vi "newRunSAS.vi"(8 "error in":errorcluster, 11 "AirSAS Controls":T1={"Receive Duration"=0.0, "I/O"={"DAQmx Device"="Dev1", "AO Range"=0.0, "AI Range"=0.0, "DAQ Group Delay"=0.0, "Fs"=0.0}, "Hardware"={"Centerpos"=[], "TXpos"=[], "RX1pos"=[], "RX2pos"=[], "Angle"=0.0, "Height"=0.0}, "Waveform"={"LFM Parameters"={"Duration"=1.0, "Fstart (Hz)"=1000.0, "Fstop (Hz)"=10000.0, "Out. Amplitude (Vpk)"=1.0, "Window %"=10.0}, "Transmit Waveform"={"t0"=timestamp(0 s since 1904-01-01), "dt"=1.0, "Y"=[]}}, "LINX Resource"={"IO"=enum."Remote", "Interface"=enum."Serial", "LINX Device Config"={"Interface"=enum."Serial", "COM Port"="COM13", "TCP Configuration"={"IP Address"="", "Port"=0}, "Device Family"=1, "Device ID"=1, "Device Name"="myRIO-1900", "TCP Ref"=refnum, "Channels"={"DI"=[0, 1, 2, 3, 4, 5, 6, 7, 8, 9, 10, 11, 12, 13, 14, 15, 16, 17, 18, 19, 20, 21, 22, 23, 24, 25, 26, 27, 28, 29, 30, 31, 32, 33, 34, 35, 36, 37, 38, 39, 40, 41, 42, 43, 44, 45, 46], "DO"=[0, 1, 2, 3, 4, 5, 6, 7, 8, 9, 10, 11, 12, 13, 14, 15, 16, 17, 18, 19, 20, 21, 22, 23, 24, 25, 26, 27, 28, 29, 30, 31, 32, 33, 34, 35, 36, 37, 38, 39, 40, 41, 42, 43, 44, 45, 46], "AI"=[0, 1, 2, 3, 4, 5, 6, 7, 8, 9, 10, 11], "AO"=[], "PWM"=[3, 5, 6, 9, 10], "QE"=[], "UART"=[0, 1], "I2C 2"=[0], "SPI"=[0], "CAN"=[], "Servo"=[], "AI Ref (V)"=0.0, "AI Resolution (Bits)"=0, "AO Ref (V)"=0.0, "AO Resolution (Bits)"=0}}}, "Port"=3000.0} {"Waveform"."LFM Parameters"."Window %" format="%.2g"; "Waveform"."LFM Parameters"."Out. Amplitude (Vpk)" format="%0.2f"; "Waveform"."LFM Parameters"."Fstop (Hz)" format="%^.3e"; "Waveform"."LFM Parameters"."Fstart (Hz)" format="%^.3e"; "Waveform"."LFM Parameters"."Duration" format="%.3f"}) -> (0 "error out":errorcluster, 3 "AirSAS Controls 2":T1={"Receive Duration"=0.0, "I/O"={"DAQmx Device"="Dev1", "AO Range"=0.0, "AI Range"=0.0, "DAQ Group Delay"=0.0, "Fs"=0.0}, "Hardware"={"Centerpos"=[], "TXpos"=[], "RX1pos"=[], "RX2pos"=[], "Angle"=0.0, "Height"=0.0}, "Waveform"={"LFM Parameters"={"Duration"=1.0, "Fstart (Hz)"=1000.0, "Fstop (Hz)"=10000.0, "Out. Amplitude (Vpk)"=1.0, "Window %"=10.0}, "Transmit Waveform"={"t0"=timestamp(0 s since 1904-01-01), "dt"=1.0, "Y"=[]}}, "LINX Resource"={"IO"=enum."Remote", "Interface"=enum."Serial", "LINX Device Config"={"Interface"=enum."Serial", "COM Port"="COM13", "TCP Configuration"={"IP Address"="", "Port"=0}, "Device Family"=1, "Device ID"=1, "Device Name"="myRIO-1900", "TCP Ref"=refnum, "Channels"={"DI"=[0, 1, 2, 3, 4, 5, 6, 7, 8, 9, 10, 11, 12, 13, 14, 15, 16, 17, 18, 19, 20, 21, 22, 23, 24, 25, 26, 27, 28, 29, 30, 31, 32, 33, 34, 35, 36, 37, 38, 39, 40, 41, 42, 43, 44, 45, 46], "DO"=[0, 1, 2, 3, 4, 5, 6, 7, 8, 9, 10, 11, 12, 13, 14, 15, 16, 17, 18, 19, 20, 21, 22, 23, 24, 25, 26, 27, 28, 29, 30, 31, 32, 33, 34, 35, 36, 37, 38, 39, 40, 41, 42, 43, 44, 45, 46], "AI"=[0, 1, 2, 3, 4, 5, 6, 7, 8, 9, 10, 11], "AO"=[], "PWM"=[3, 5, 6, 9, 10], "QE"=[], "UART"=[0, 1], "I2C 2"=[0], "SPI"=[0], "CAN"=[], "Servo"=[], "AI Ref (V)"=0.0, "AI Resolution (Bits)"=0, "AO Ref (V)"=0.0, "AO Resolution (Bits)"=0}}}, "Port"=3000.0} {"Waveform"."LFM Parameters"."Window %" format="%.2g"; "Waveform"."LFM Parameters"."Out. Amplitude (Vpk)" format="%0.2f"; "Waveform"."LFM Parameters"."Fstop (Hz)" format="%^.3e"; "Waveform"."LFM Parameters"."Fstart (Hz)" format="%^.3e"; "Waveform"."LFM Parameters"."Duration" format="%.3f"})   [LabVIEW 2018]
uses:
  N:/SRDD-Student/Ng/fromTom/Air SAS Data Acquisition/controls/Air SAS Controls.ctl
  <vilib>/MakerHub/LINX/Private/Type Defs/LINX Ref.ctl
  <vilib>/MakerHub/LINX/Private/Type Defs/Platform.ctl
  <vilib>/MakerHub/LINX/Private/Type Defs/Interface.ctl
  <vilib>/MakerHub/LINX/Private/Device/Type Defs/LINX Device Config.ctl
  <vilib>/MakerHub/LINX/Private/Device/Type Defs/TCP Config.ctl
  <vilib>/MakerHub/LINX/Private/Device/Type Defs/Channels.ctl
  <vilib>/Analysis/4window.llb/Cosine Tapered Window (DBL).vi
  <vilib>/Waveform/WDTOps.llb/WDT Number of Waveform Samples DBL.vi
  <vilib>/regexp/Match Regular Expression.xnode
  <vilib>/Analysis/NI_AALBase.lvlib
  <vilib>/Analysis/NI_AALPro.lvlib
  <vilib>/MakerHub/LINX/LMH-LINX.lvlib
  <vilib>/MakerHub/LINX/Private/Device/Device.lvlib
panel:
  in  "Folder Path":path=path "C:/Users/jqn5303/Desktop/testfiles"
  in  "stop":bool
  out "Transmit Waveform":waveform(dbl)(graph)
  in  "LFM Parameters":T8={"Fs (Hz)"=100000.0, "Sweep Length (s)"=0.001, "Fstart (Hz)"=10000.0, "Fstop (Hz)"=10000.0, "Out. Amplitude (Vpk)"=1.0, "Window %"=10.0} {"Window %" format="%.2g"; "Out. Amplitude (Vpk)" format="%0.2f"; "Fstop (Hz)" format="%^.3e"; "Fstart (Hz)" format="%^.3e"; "Sweep Length (s)" format="%.3f"; "Fs (Hz)" min=1000.0 max=2000000.0 format="%^.0e"}
  in  "Generate LFM":bool
  in  "Start Acquisition":bool
  out "Acquired Data":waveform(dbl)(graph)
  out "Slide":cluster{dbl, dbl, dbl}(slide)={0.0, 227.2365805168986, 42.94234592445328} scale=0.0..900.0
  out "Gauge":cluster{dbl, dbl, dbl}(knob)={0.0, -178.0803549193409, -96.36742372843878} scale format="%#_g°"
  in  "Motion Control":T9={"SAS Geometry"=enum."Circular", "Angular Step"=1.0, "Vertical Step"=0.0, "Vertical Min"=0.0, "Vertical Max"=0.0, "Angular Start"=0.0, "Angular Stop"=359.0}
  in  "Receive Duration":dbl=0.01
  in  "Averages":dbl=1.0 min=1.0 step=1.0
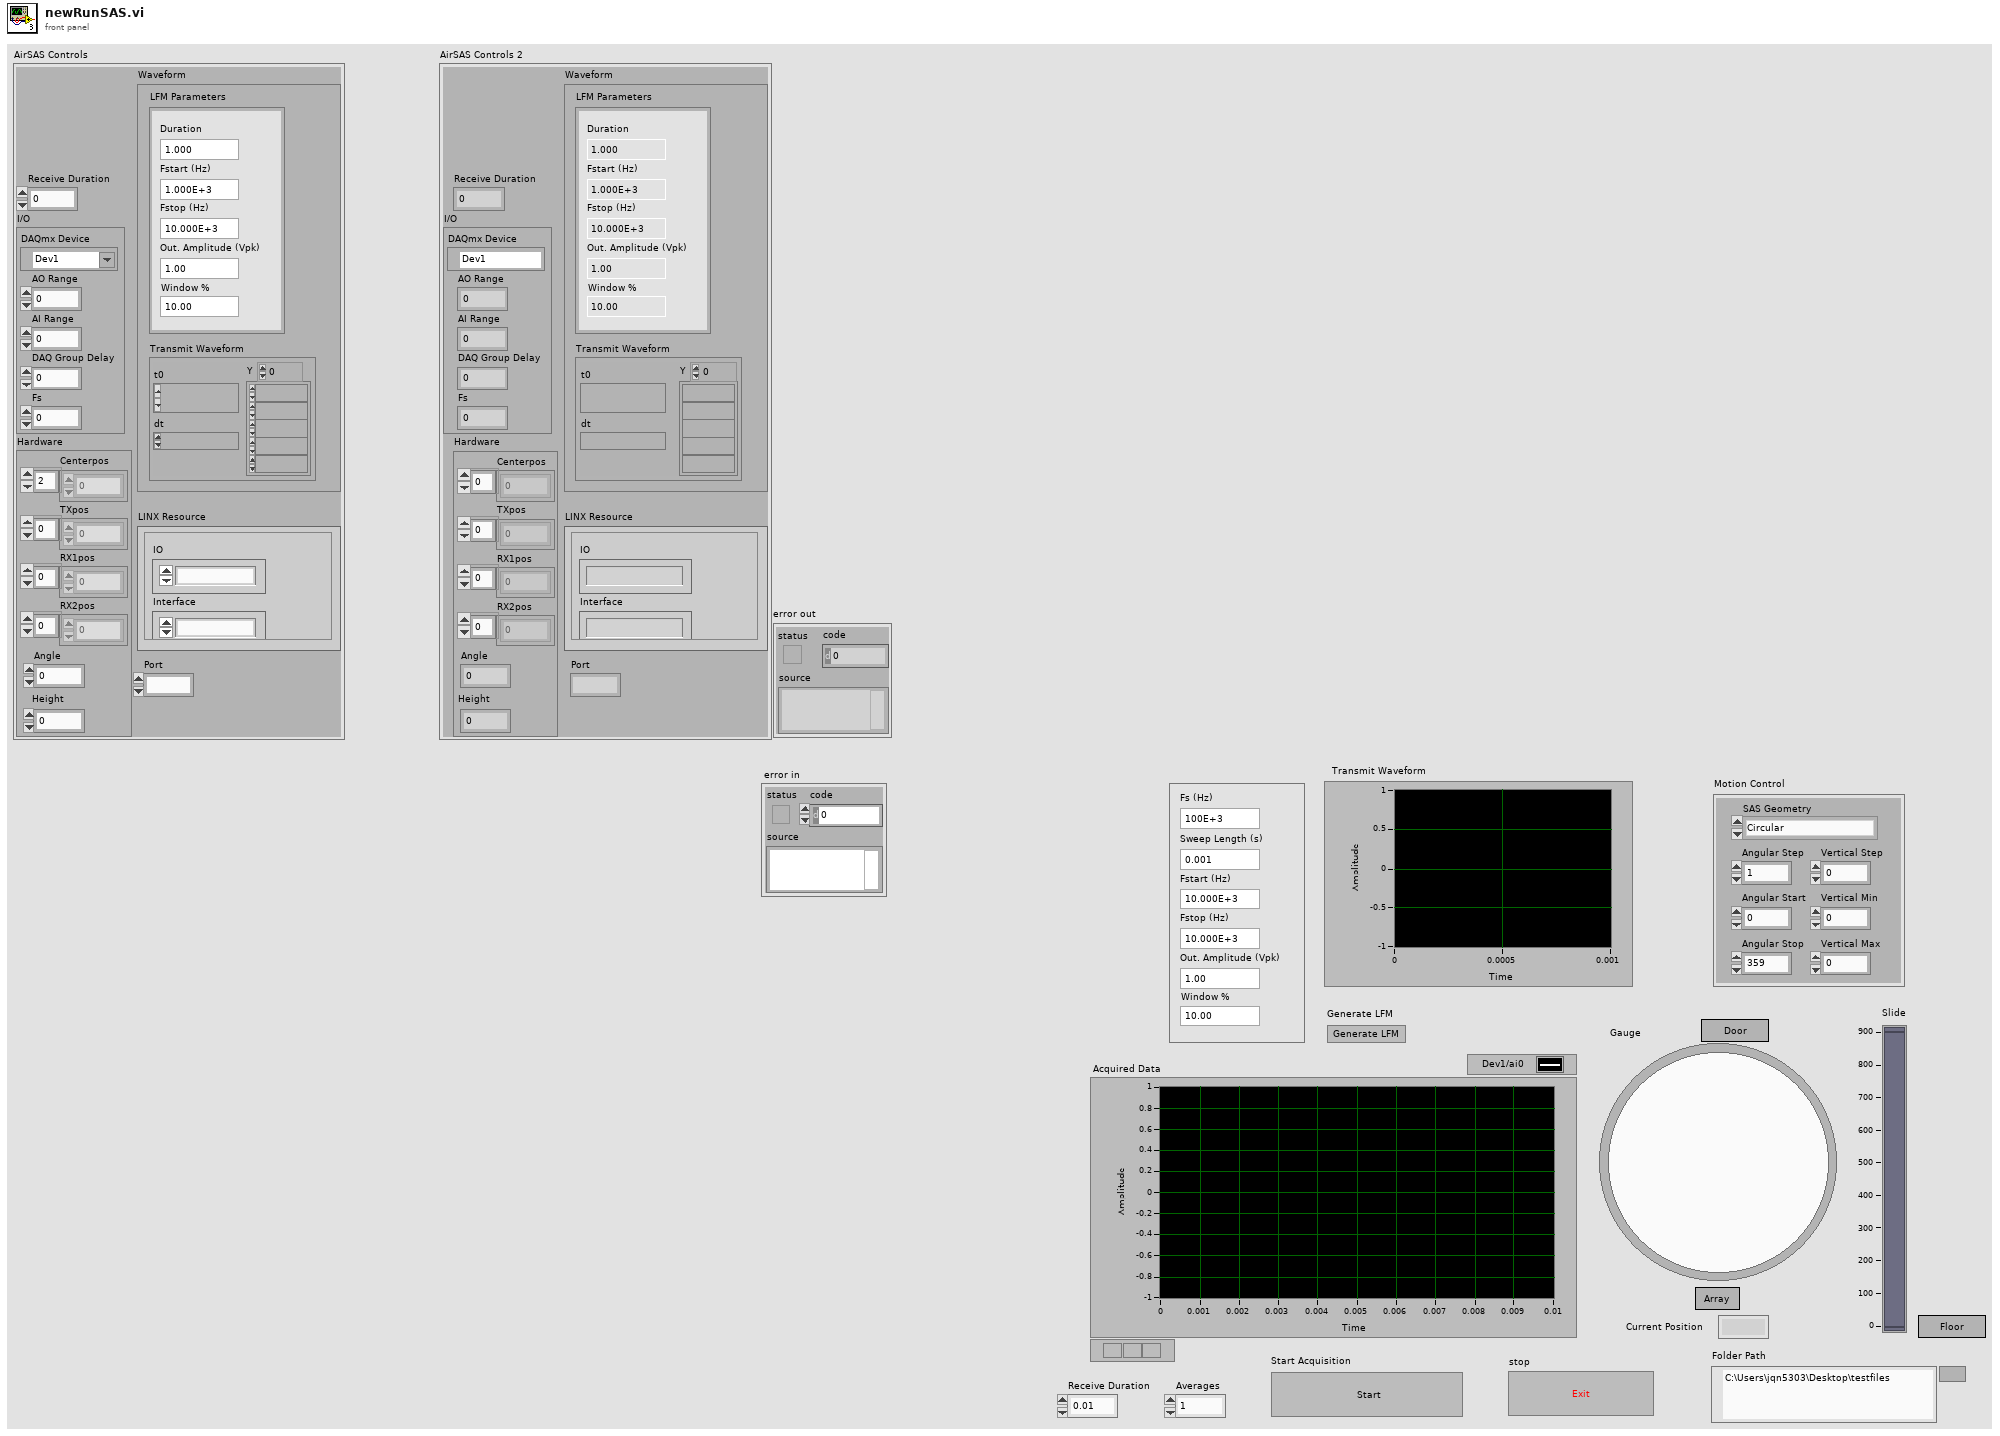
[diagram p1: front panel]
types:
  T1 = typedef "Air SAS Controls.ctl" = cluster{"Receive Duration":dbl, "I/O":cluster{"DAQmx Device":tag, "AO Range":dbl, "AI Range":dbl, "DAQ Group Delay":dbl, "Fs":dbl}, "Hardware":cluster{"Centerpos":dbl[], "TXpos":dbl[], "RX1pos":dbl[], "RX2pos":dbl[], "Angle":dbl, "Height":dbl}, "Waveform":cluster{"LFM Parameters":cluster{"Duration":dbl, "Fstart (Hz)":dbl, "Fstop (Hz)":dbl, "Out. Amplitude (Vpk)":dbl, "Window %":dbl}, "Transmit Waveform":waveform(dbl)}, "LINX Resource":T2, "Port":dbl}
  T2 = typedef "LMH-LINX.lvlib/LINX Ref.ctl" = cluster{"IO":T3, "Interface":T4, "LINX Device Config":T5}
  T3 = typedef "LMH-LINX.lvlib/Platform.ctl" = enum16{"Remote", "Local"}
  T4 = typedef "LMH-LINX.lvlib/Interface.ctl" = enum16{"Serial", "TCP"}
  T5 = typedef "LMH-LINX.lvlib/Device.lvlib/LINX Device Config.ctl" = cluster{"Interface":T4, "COM Port":refnum<visa-resource-name>, "TCP Configuration":T6, "Device Family":u8, "Device ID":u8, "Device Name":string, "TCP Ref":refnum<k5>, "Channels":T7}
  T6 = typedef "LMH-LINX.lvlib/Device.lvlib/TCP Config.ctl" = cluster{"IP Address":string, "Port":u16}
  T7 = typedef "LMH-LINX.lvlib/Channels.ctl" = cluster{"DI":u8[], "DO":u8[], "AI":u8[], "AO":u8[], "PWM":u8[], "QE":u8[], "UART":u8[], "I2C 2":u8[], "SPI":u8[], "CAN":u8[], "Servo":u8[], "AI Ref (V)":dbl, "AI Resolution (Bits)":u8, "AO Ref (V)":dbl, "AO Resolution (Bits)":u8}
  T8 = cluster{"Fs (Hz)":dbl, "Sweep Length (s)":dbl, "Fstart (Hz)":dbl, "Fstop (Hz)":dbl, "Out. Amplitude (Vpk)":dbl, "Window %":dbl}
  T9 = cluster{"SAS Geometry":enum16{"Circular", "Cylindrical", "Spiral"}, "Angular Step":dbl, "Vertical Step":dbl, "Vertical Min":dbl, "Vertical Max":dbl, "Angular Start":dbl, "Angular Stop":dbl}
  T10 = enum8{"Enabled", "Disabled", "Disabled and Grayed Out"}
  T11 = cluster{"Angular Start":dbl, dbl, "Angular Stop":dbl}
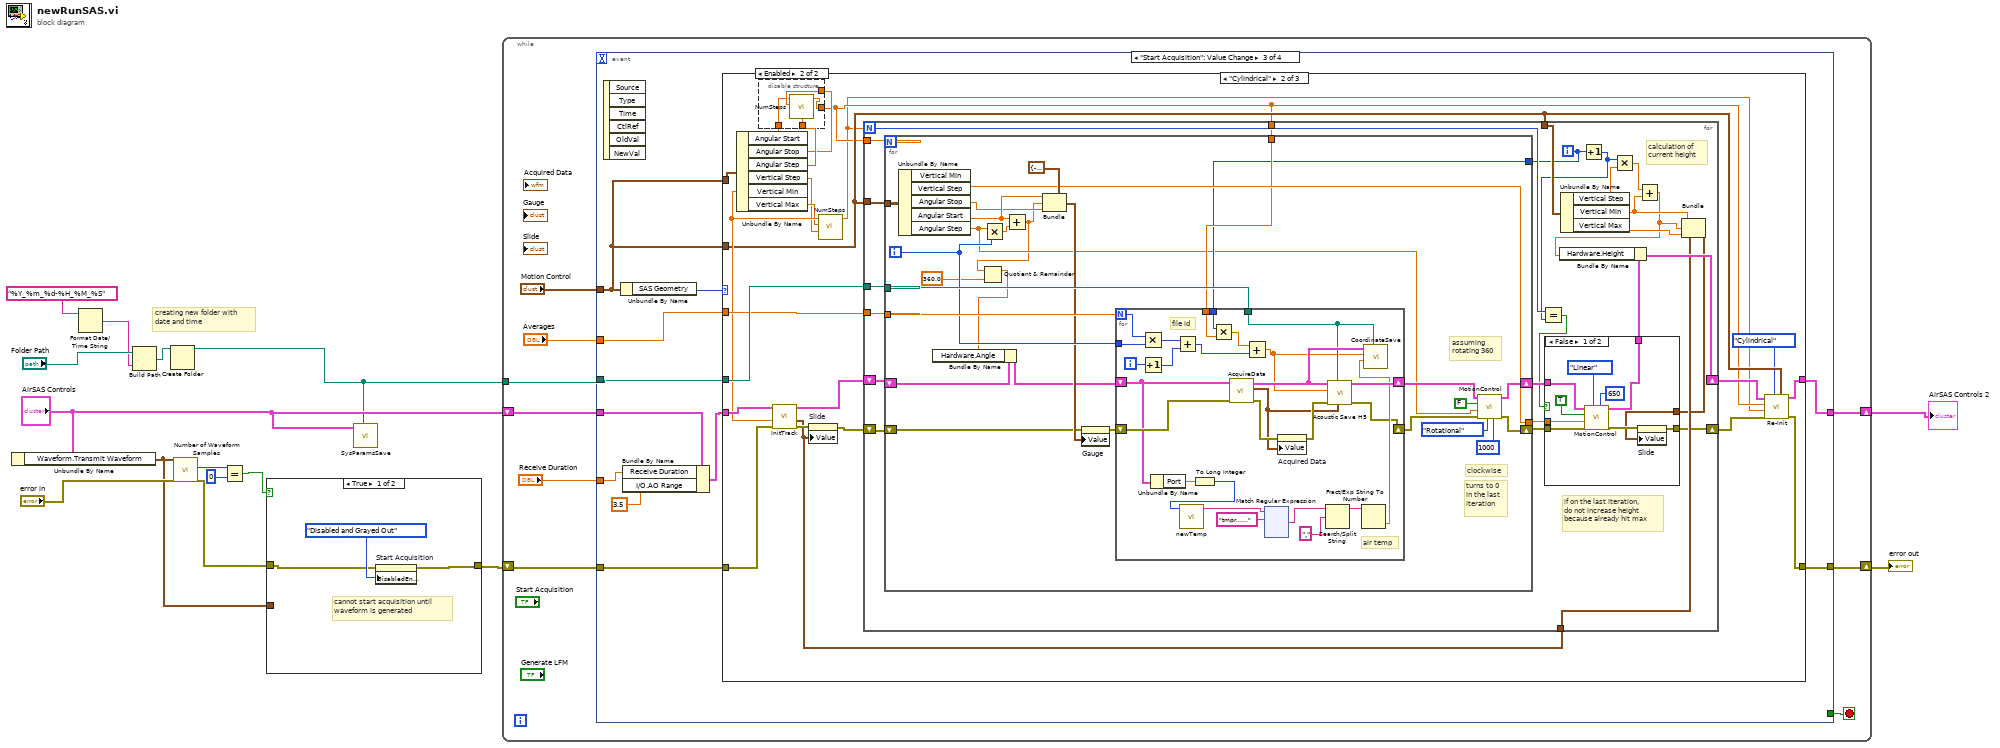
[diagram p0: block diagram]
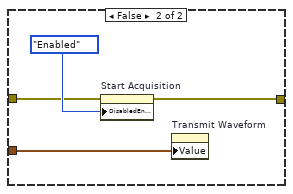
[diagram p2: hidden frame]
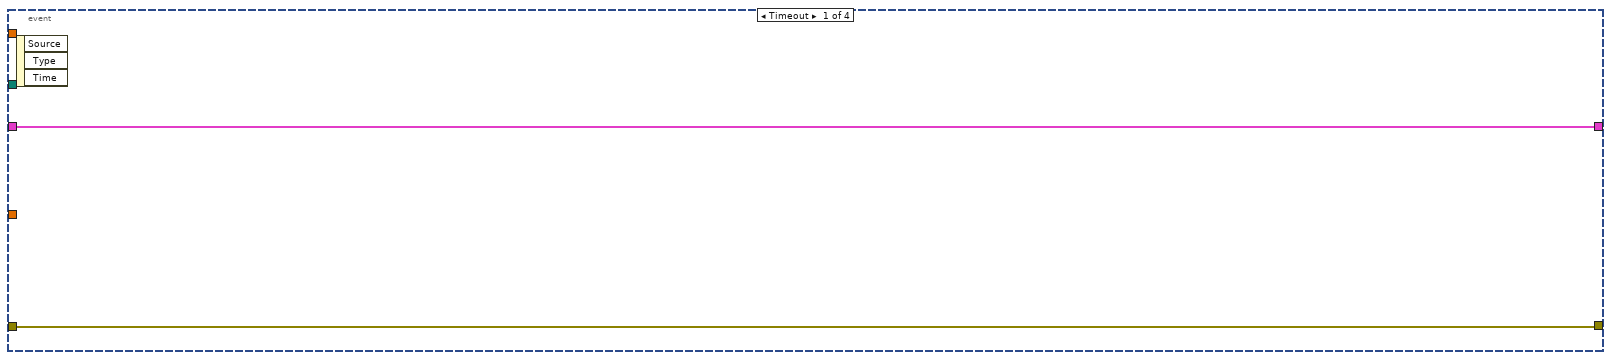
[diagram p3: hidden frame]
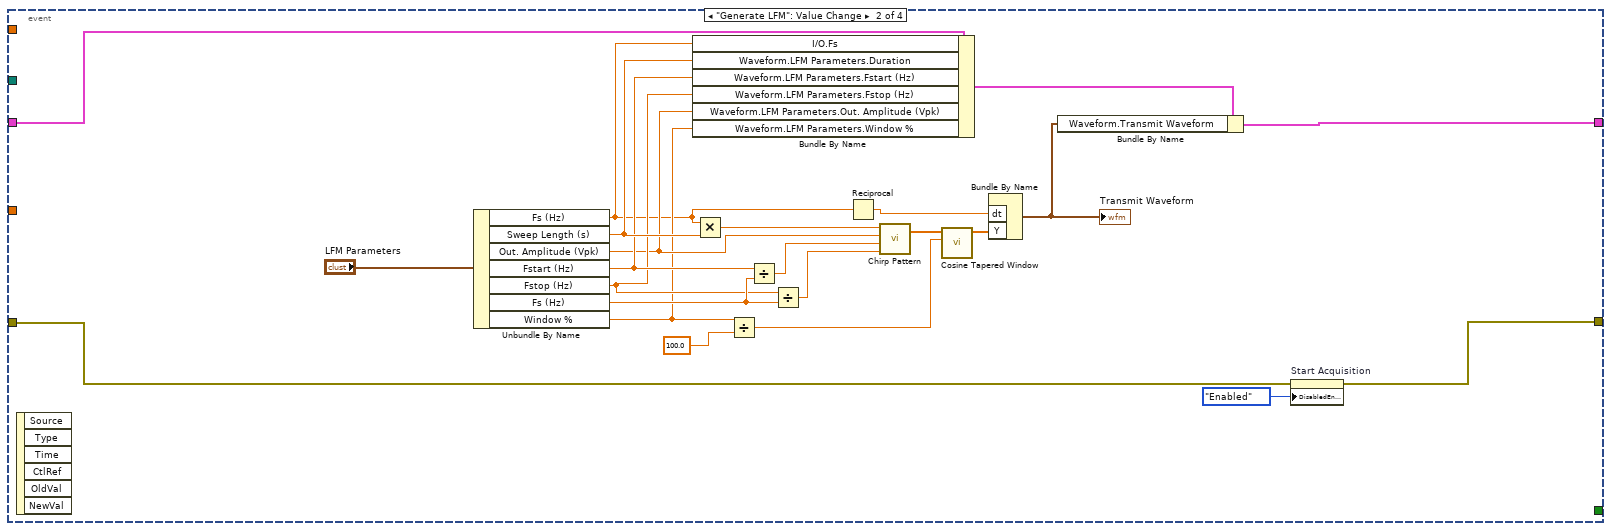
[diagram p4: hidden frame]
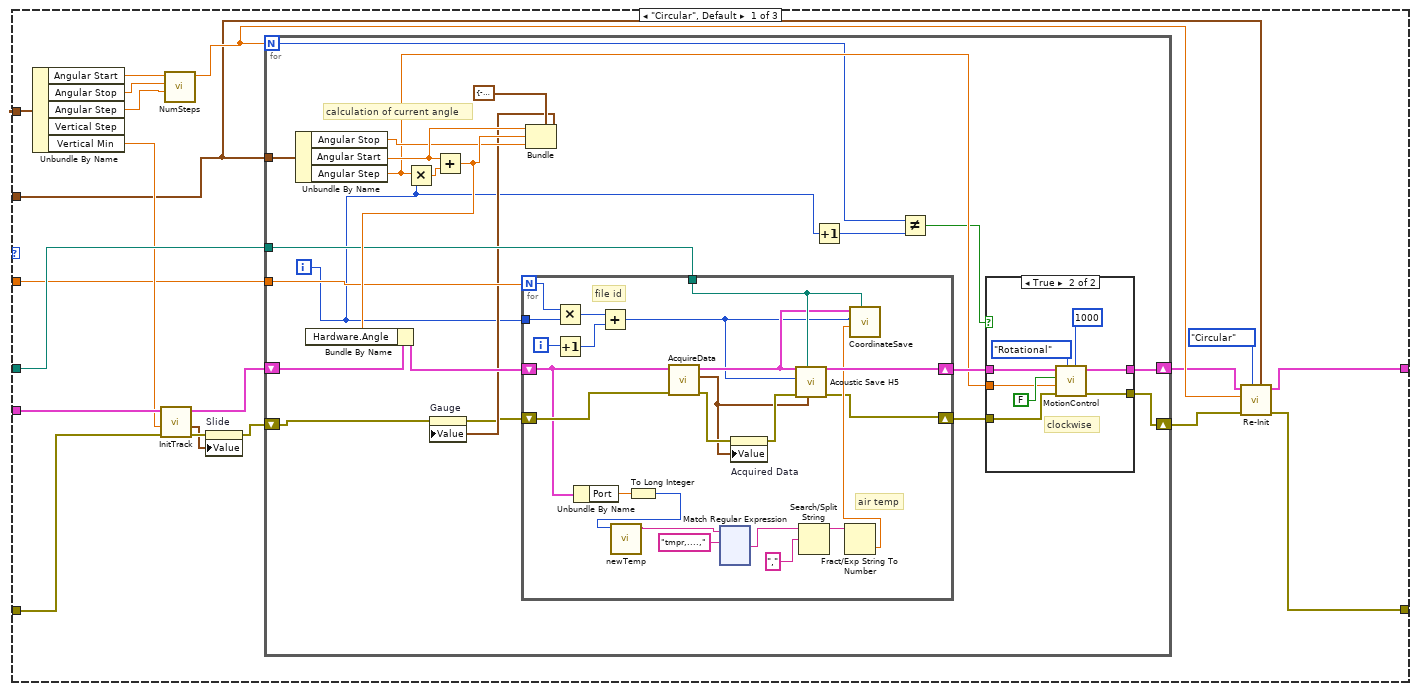
[diagram p5: hidden frame]
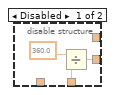
[diagram p7: hidden frame]
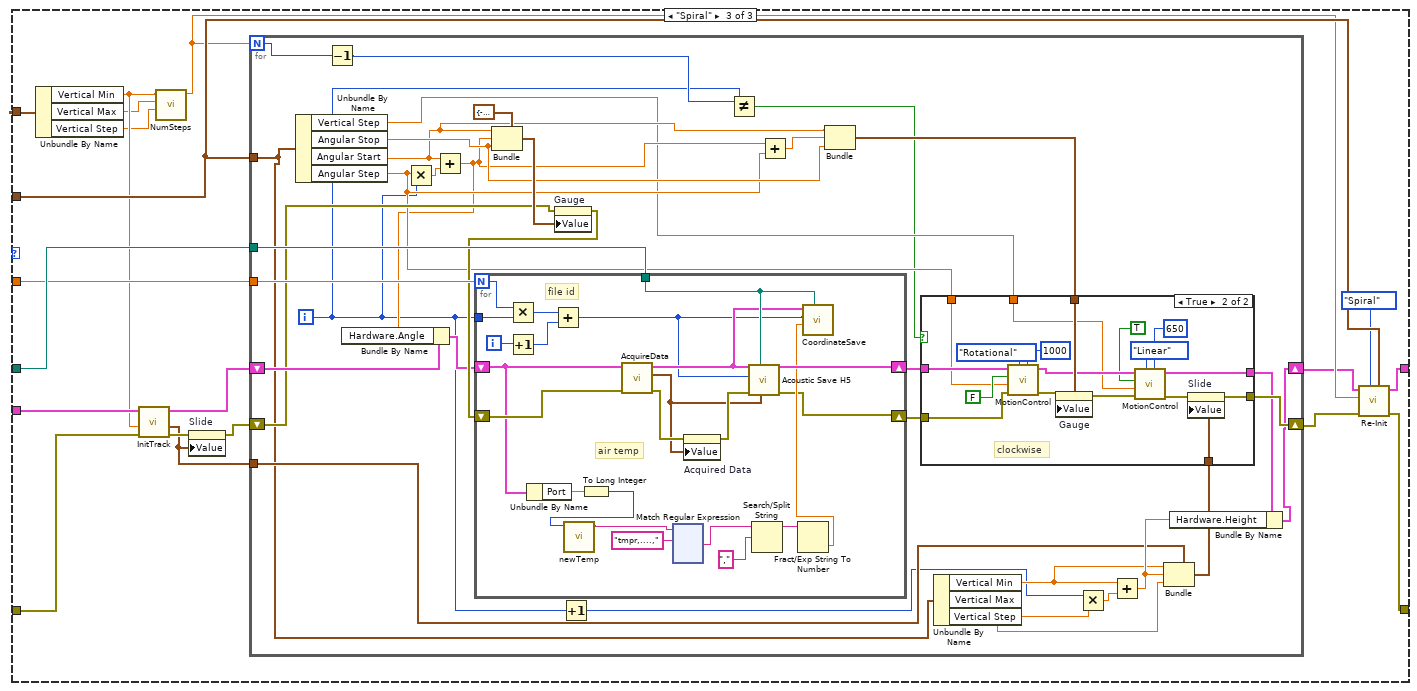
[diagram p9: hidden frame]
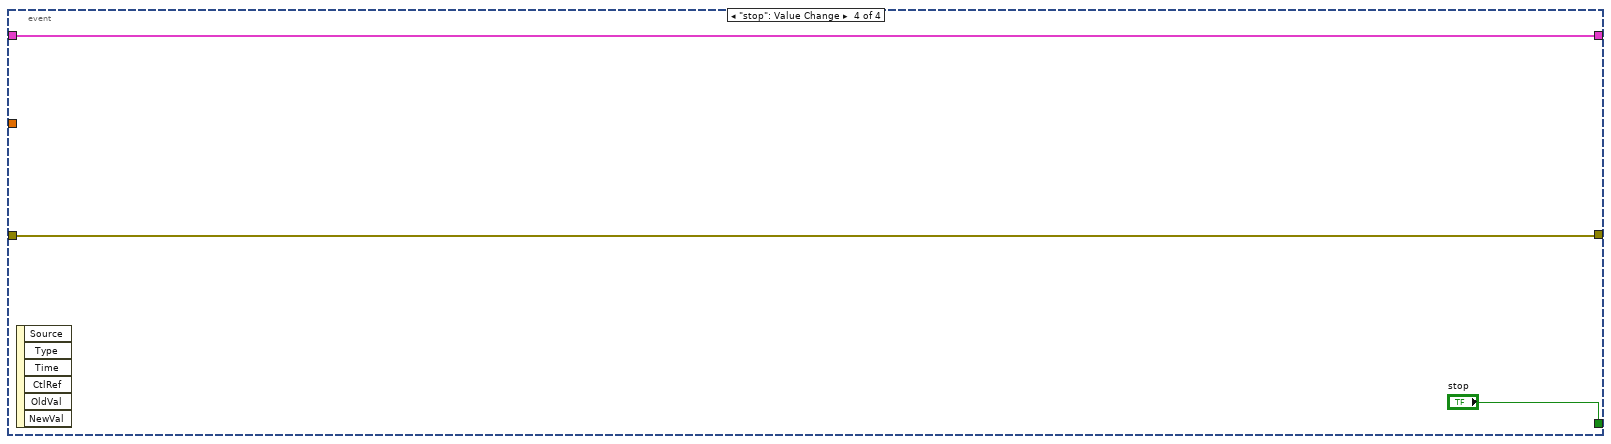
[diagram p11: hidden frame]
diagram:
  # "creating new folder with\ndate and time"
  n1 = Unbundle By Name("AirSAS Controls") -> ("Waveform.Transmit Waveform"=w8:waveform(dbl))
  n2 = Format Date/Time String(time format string (%c)="%Y_%m_%d-%H_%M_%S") -> (date/time string=w3:string)  [unwired: 2 in]
  n3 = Build Path(base path="Folder Path", name or relative path=w3) -> (appended path=w2:path)
  n4 = Create Folder(path (use dialog)=w2) -> (created path=w1:path)  [unwired: 2 in, 2 out]
  n5 = call-poly <vilib>:"Number of Waveform Samples.vi"("error in (no error)"="error in", "waveform in"=w8) -> ("error out"=w9:errorcluster, "number of samples"=w14:i32)  [unwired: 7 in, 1 out]
  n6 = Equal?(x=w14, y=0) -> (x = y?=w12:bool)
  n7 = case shown="True" w12 {
    tunnel: [w16 w20] -> w10
    tunnel: w9 -> [w17 w19]
    tunnel: w8 -> [_ w21]
    frame True {
      # "cannot start acquisition until\nwaveform is generated"
      n8 = property on="Start Acquisition" class="Bool"(error in=w17, "DisabledEnum"=T10."Disabled and Grayed Out" ("Disabled")) -> (error out=w16:errorcluster)  [unwired: 1 in, 1 out]
    }
    frame False {
      n9 = property on="Start Acquisition" class="Bool"(error in=w19, "DisabledEnum"=T10."Enabled" ("Disabled")) -> (error out=w20:errorcluster)  [unwired: 1 in, 1 out]
      n10 = property on="Transmit Waveform" class="WFGraph (strict)"("Value"=w21) -> ()  [unwired: 2 in, 2 out]
    }
  }
  n11 = call "SysParamsSave.vi"("Path"=w1, "AirSAS Controls"="AirSAS Controls") -> ()  [unwired: 10 in]
  n12 = while {
    shift-right: [w30] -> w7
    shift-left: "AirSAS Controls" -> [w31]
    shift-right: [w27] -> w15
    shift-left: w10 -> [w28]
    tunnel: w1 -> [w26]
    stop <- w29 stop-if-true
    n13 = event shown="[2] \"Start Acquisition\": Value Change" {
      selector: _ -> [_ _ _ _]
      dyn-events: _ -> [_ _ _ _]
      timeout: _ -> [_ _ _ _]
      tunnel: w31 -> [w33 w46 w64 w700]
      tunnel: [w33 w38 w59 w700] -> w30
      tunnel: [_ _ _ "stop"] -> w29
      tunnel: w28 -> [w32 w35 w63 w699]
      tunnel: [w32 w34 w58 w699] -> w27
      tunnel: w26 -> [_ _ w61 _]
      tunnel: "Motion Control" -> [_ _ w62 _]
      tunnel: "Receive Duration" -> [_ _ w66 _]
      tunnel: "Averages" -> [_ _ w60 _]
      event Timeout {
        n14 = event-data() -> ()  [unwired: 1 in, 3 out]
      }
      event "Generate LFM": Value Change {
        n15 = event-data() -> ()  [unwired: 1 in, 6 out]
        n16 = Unbundle By Name("LFM Parameters") -> ("Fs (Hz)"=w37:dbl, "Sweep Length (s)"=w45:dbl, "Out. Amplitude (Vpk)"=w42:dbl, "Fstart (Hz)"=w44:dbl, "Fstop (Hz)"=w43:dbl, "Fs (Hz)"=w54:dbl, "Window %"=w41:dbl)
        n17 = Bundle By Name(cluster=w46, "I/O.Fs"=w37, "Waveform.LFM Parameters.Duration"=w45, "Waveform.LFM Parameters.Fstart (Hz)"=w44, "Waveform.LFM Parameters.Fstop (Hz)"=w43, "Waveform.LFM Parameters.Out. Amplitude (Vpk)"=w42, "Waveform.LFM Parameters.Window %"=w41) -> (w40:T1)
        n18 = Multiply(x=w37, y=w45) -> (x*y=w56:dbl)
        n19 = Divide(x=w41, y=100.0) -> (x/y=w49:dbl)
        n20 = Divide(x=w44, y=w54) -> (x/y=w55:dbl)
        n21 = Divide(x=w43, y=w54) -> (x/y=w53:dbl)
        n22 = Reciprocal(x=w37) -> (1/x=w50:dbl)
        n23 = call <vilib>:"Chirp Pattern.vi"("f2"=w53, "f1"=w55, "amplitude"=w42, "samples"=w56) -> ("Chirp Pattern"=w52:dbl[])  [unwired: 1 out]
        n24 = call-poly <vilib>:"Cosine Tapered Window.vi"("ratio"=w49, "X"=w52) -> ("Windowed X"=w51:dbl[])  [unwired: 8 in, 1 out]
        n25 = Bundle By Name("dt"=w50, "Y"=w51) -> (w39:waveform(dbl))  [unwired: 1 in]
        "Transmit Waveform" <- w39
        n26 = Bundle By Name(cluster=w40, "Waveform.Transmit Waveform"=w39) -> (w38:T1)
        n27 = property on="Start Acquisition" class="Bool"(error in=w35, "DisabledEnum"=T10."Enabled" ("Disabled")) -> (error out=w34:errorcluster)  [unwired: 1 in, 1 out]
      }
      event "Start Acquisition": Value Change {
        n28 = event-data() -> ()  [unwired: 1 in, 6 out]
        n29 = Unbundle By Name(w62) -> ("SAS Geometry"=w67:enum16{"Circular", "Cylindrical", "Spiral"})
        n30 = Bundle By Name(cluster=w64, "Receive Duration"=w66, "I/O.AO Range"=3.5) -> (w57:T1)
        n31 = case shown="\"Cylindrical\"" w67 {
          tunnel: w62 -> [w87 w278 w508]
          tunnel: w57 -> [w85 w276 w506]
          tunnel: w63 -> [w83 w275 w505]
          tunnel: w62 -> [w76 w261 w500]
          tunnel: w61 -> [w86 w277 w507]
          tunnel: [w72 w262 w491] -> w59
          tunnel: w60 -> [w81 w273 w503]
          tunnel: [w74 w259 w498] -> w58
          frame "Circular", Default {
            n32 = Unbundle By Name(w87) -> ("Angular Start"=w71:dbl, "Angular Stop"=w70:dbl, "Angular Step"=w69:dbl, "Vertical Min"=w84:dbl)  [unwired: 1 out]
            n33 = call "InitTrack.vi"("AirSAS Controls in"=w85, "Vertical Min"=w84, "error in (no error)"=w83) -> ("AirSAS Controls out"=w82:T1, "output cluster"=w78:cluster{dbl, dbl, dbl}, "error out"=w80:errorcluster)  [unwired: 4 in]
            n34 = call "NumSteps.vi"("Step"=w69, "Stop"=w70, "Start"=w71) -> ("Numeric"=w77:dbl)  [unwired: 8 in]
            n35 = property on="Slide" class="Slide (strict)"(error in=w80, "Value"=w78) -> (error out=w79:errorcluster)  [unwired: 1 in, 1 out]
            n36 = for {
              N: w77 -> [w88]
              tunnel: w76 -> [w109]
              tunnel: w86 -> [w102]
              shift-right: [w98] -> w73
              shift-left: w82 -> [w108]
              tunnel: w81 -> [w101]
              shift-right: [w93] -> w75
              shift-left: w79 -> [w95]
              i -> [w89]
              # "calculation of current angle"
              n37 = Unbundle By Name(w109) -> ("Angular Stop"=w104:dbl, "Angular Start"=w106:dbl, "Angular Step"=w97:dbl)
              n38 = Multiply(x=w97, y=w89) -> (x*y=w107:dbl)
              n39 = Add(x=w106, y=w107) -> (x+y=w105:dbl)
              n40 = Bundle By Name(cluster=w108, "Hardware.Angle"=w105) -> (w100:T1)
              n41 = Bundle(cluster=cluster{dbl, dbl, dbl} {-172.55422153679154, 17.21837893351085, -51.118830131082746} ("Gauge 2"), w106, w105, w104) -> (w96:cluster{dbl, dbl, dbl})
              n42 = property on="Gauge" class="Knob (strict)"(error in=w95, "Value"=w96) -> (error out=w94:errorcluster)  [unwired: 1 in, 1 out]
              n43 = for {
                N: w101 -> [w139]
                tunnel: w89 -> [w138]
                tunnel: w102 -> [w124]
                shift-right: [w123] -> w99
                shift-left: w100 -> [w125]
                shift-right: [w120] -> w92
                shift-left: w94 -> [w136]
                i -> [w137]
                # "air temp"
                # "file id"
                n44 = Multiply(x=w139, y=w138) -> (x*y=w141:i32)
                n45 = Increment(x=w137) -> (x+1=w140:i32)
                n46 = Unbundle By Name(w125) -> ("Port"=w131:dbl)
                n47 = Add(x=w141, y=w140) -> (x+y=w122:i32)
                n48 = To Long Integer(number=w131) -> (32bit integer=w132:i32)
                n49 = call "newTemp.vi"("port"=w132) -> ("Response String"=w130:string)  [unwired: 10 in]
                n50 = call "AcquireData.vi"("error in"=w136, "AirSAS Controls In"=w125) -> ("error out"=w135:errorcluster, "data"=w133:waveform(dbl), "AirSAS Controls Out"=w123:T1)  [unwired: 7 in]
                n51 = xnode "Match Regular Expression"("input string"=w130, "regular expression"="tmpr,....,") -> ("after match"=w128:string)  [unwired: 4 in, 4 out]
                n52 = property on="Acquired Data" class="WFGraph (strict)"(error in=w135, "Value"=w133) -> (error out=w134:errorcluster)  [unwired: 1 in, 1 out]
                n53 = call "Acoustic Save H5.vi"("Captured Data"=w133, "base path"=w124, "error in (no error)"=w134, "ID"=w122) -> ("error out"=w120:errorcluster)  [unwired: 7 in]
                n54 = Search/Split String(string=w128, search string/char (-)=",") -> (substring before match=w129:string)  [unwired: 1 in, 2 out]
                n55 = Fract/Exp String To Number(string=w129) -> (number=w121:dbl)  [unwired: 3 in, 1 out]
                n56 = call "CoordinateSave.vi"("Path"=w124, "Air Temperature"=w121, "Flight"=w122, "AirSAS Controls"=w123) -> ()  [unwired: 8 in]
              }
              n57 = Increment(x=w89) -> (x+1=w90:i32)
              n58 = Not Equal?(x=w88, y=w90) -> (x != y?=w91:bool)
              n59 = case shown="True" w91 {
                tunnel: w99 -> [w111 w117]
                tunnel: [w111 w116] -> w98
                tunnel: w97 -> [_ w114]
                tunnel: [w110 w113] -> w93
                tunnel: w92 -> [w110 w112]
                frame False {
                }
                frame True {
                  # "clockwise"
                  n60 = call "MotionControl.vi"("Frequency (Hz) 3"=u32 1000, "Motion Type"=enum16{"Linear", "Rotational"}."Rotational", "Error In"=w112, "Distance"=w114, "Direction"=FALSE, "AirSAS Controls"=w117) -> ("Error Out"=w113:errorcluster, "output cluster"=w116:T1)  [unwired: 4 in]
                }
              }
            }
            n61 = call "Re-Init.vi"("Motion Control"=w76, "Enum"=enum16{"Circular", "Cylindrical", "Spiral"}."Circular", "error in (no error)"=w75, "# rot. steps"=w77, "AirSAS Controls"=w73) -> ("error out"=w74:errorcluster, "output cluster"=w72:T1)  [unwired: 5 in]
          }
          frame "Cylindrical" {
            n62 = Unbundle By Name(w278) -> ("Angular Start"=w264:dbl, "Angular Stop"=w265:dbl, "Angular Step"=w272:dbl, "Vertical Step"=w266:dbl, "Vertical Min"=w268:dbl, "Vertical Max"=w267:dbl)
            n63 = disable-structure shown="Enabled" {
              disable-tunnel: w272 -> [w280 w285]
              disable-tunnel: [w279 w282] -> w258
              disable-tunnel: w265 -> [_ w284]
              disable-tunnel: w264 -> [_ w283]
              frame Disabled {
                n64 = Divide(x=360.0, y=w280) -> (x/y=w279:dbl)
              }
              frame Enabled {
                n65 = call "NumSteps.vi"("Step"=w285, "Stop"=w284, "Start"=w283) -> ("Numeric"=w282:dbl)  [unwired: 8 in]
              }
            }
            n66 = call "InitTrack.vi"("AirSAS Controls in"=w276, "Vertical Min"=w268, "error in (no error)"=w275) -> ("AirSAS Controls out"=w274:T1, "output cluster"=w269:cluster{dbl, dbl, dbl}, "error out"=w271:errorcluster)  [unwired: 4 in]
            n67 = property on="Slide" class="Slide (strict)"(error in=w271, "Value"=w269) -> (error out=w270:errorcluster)  [unwired: 1 in, 1 out]
            n68 = call "NumSteps.vi"("Step"=w266, "Stop"=w267, "Start"=w268) -> ("Numeric"=w257:dbl)  [unwired: 8 in]
            n69 = for {
              N: w257 -> [w290]
              tunnel: w261 -> [w310]
              tunnel: w277 -> [w307]
              shift-right: [w299] -> w263
              shift-left: w274 -> [w309]
              tunnel: w273 -> [w306]
              tunnel: w258 -> [w305]
              tunnel: w261 -> [w302]
              tunnel: w269 -> [w298]
              shift-right: [w294] -> w260
              shift-left: w270 -> [w308]
              tunnel: w258 -> [w287]
              i -> [w286]
              # "if on the last iteration,\ndo not increase height\nbecause already hit max"
              # "calculation of\ncurrent height"
              n70 = for {
                N: w305 -> [_]
                tunnel: w310 -> [w349]
                tunnel: w307 -> [w343]
                tunnel: w306 -> [w342]
                shift-right: [w327] -> w293
                shift-left: w309 -> [w348]
                shift-right: [w329] -> w304
                shift-left: w308 -> [w334]
                tunnel: [w340] -> w303
                tunnel: w287 -> [w338]
                tunnel: w286 -> [w337]
                i -> [w339]
                # "assuming\nrotating 360"
                # "turns to 0\nin the last\niteration"
                # "clockwise"
                n71 = Unbundle By Name(w349) -> ("Vertical Step"=w340:dbl, "Angular Stop"=w345:dbl, "Angular Start"=w346:dbl, "Angular Step"=w326:dbl)  [unwired: 1 out]
                n72 = Multiply(x=w326, y=w339) -> (x*y=w347:dbl)
                n73 = Add(x=w346, y=w347) -> (x+y=w325:dbl)
                n74 = Quotient & Remainder(x=w325, y=360.0) -> (x-y*floor(x/y)=w323:dbl)  [unwired: 1 out]
                n75 = Bundle By Name(cluster=w348, "Hardware.Angle"=w323) -> (w335:T1)
                n76 = Bundle(cluster=cluster{dbl, dbl, dbl} {-172.55422153679154, 17.21837893351085, -51.118830131082746} ("Gauge 2"), w346, w325, w345) -> (w336:cluster{dbl, dbl, dbl})
                n77 = property on="Gauge" class="Knob (strict)"(error in=w334, "Value"=w336) -> (error out=w341:errorcluster)  [unwired: 1 in, 1 out]
                n78 = for {
                  N: w342 -> [w373]
                  tunnel: w339 -> [w372]
                  tunnel: w343 -> [w356]
                  shift-right: [w358] -> w328
                  shift-left: w335 -> [w359]
                  shift-right: [w350] -> w330
                  shift-left: w341 -> [w370]
                  tunnel: w337 -> [w355]
                  tunnel: w338 -> [w354]
                  i -> [w371]
                  # "air temp"
                  # "file id"
                  n79 = Multiply(x=w373, y=w372) -> (x*y=w375:i32)
                  n80 = Increment(x=w371) -> (x+1=w374:i32)
                  n81 = Unbundle By Name(w359) -> ("Port"=w361:dbl)
                  n82 = Add(x=w375, y=w374) -> (x+y=w353:i32)
                  n83 = To Long Integer(number=w361) -> (32bit integer=w360:i32)
                  n84 = call "newTemp.vi"("port"=w360) -> ("Response String"=w362:string)  [unwired: 10 in]
                  n85 = Multiply(x=w355, y=w354) -> (x*y=w352:dbl)
                  n86 = call "AcquireData.vi"("error in"=w370, "AirSAS Controls In"=w359) -> ("error out"=w369:errorcluster, "data"=w367:waveform(dbl), "AirSAS Controls Out"=w358:T1)  [unwired: 7 in]
                  n87 = Add(x=w352, y=w353) -> (x+y=w351:dbl)
                  n88 = xnode "Match Regular Expression"("input string"=w362, "regular expression"="tmpr,....,") -> ("after match"=w364:string)  [unwired: 4 in, 4 out]
                  n89 = property on="Acquired Data" class="WFGraph (strict)"(error in=w369, "Value"=w367) -> (error out=w368:errorcluster)  [unwired: 1 in, 1 out]
                  n90 = Search/Split String(string=w364, search string/char (-)=",") -> (substring before match=w363:string)  [unwired: 1 in, 2 out]
                  n91 = call "Acoustic Save H5.vi"("Captured Data"=w367, "base path"=w356, "error in (no error)"=w368, "ID"=w351) -> ("error out"=w350:errorcluster)  [unwired: 7 in]
                  n92 = Fract/Exp String To Number(string=w363) -> (number=w357:dbl)  [unwired: 3 in, 1 out]
                  n93 = call "CoordinateSave.vi"("Path"=w356, "Air Temperature"=w357, "Flight"=w351, "AirSAS Controls"=w358) -> ()  [unwired: 8 in]
                }
                n94 = call "MotionControl.vi"("Frequency (Hz) 3"=u32 1000, "Motion Type"=enum16{"Linear", "Rotational"}."Rotational", "Error In"=w330, "Distance"=w326, "Direction"=FALSE, "AirSAS Controls"=w328) -> ("Error Out"=w329:errorcluster, "output cluster"=w327:T1)  [unwired: 4 in]
              }
              n95 = Unbundle By Name(w302) -> ("Vertical Step"=w301:dbl, "Vertical Min"=w297:dbl, "Vertical Max"=w296:dbl)
              n96 = Increment(x=w286) -> (x+1=w288:i32)
              n97 = Equal?(x=w290, y=w288) -> (x = y?=w289:bool)
              n98 = Multiply(x=w288, y=w301) -> (x*y=w300:dbl)
              n99 = Add(x=w300, y=w297) -> (x+y=w291:dbl)
              n100 = Bundle(cluster=w298, w297, w291, w296) -> (w295:cluster{dbl, dbl, dbl})
              n101 = case shown="False" w289 {
                tunnel: w304 -> [w320 w321]
                tunnel: w303 -> [w317 _]
                tunnel: w295 -> [w315 _]
                tunnel: [w314 w321] -> w294
                tunnel: w293 -> [w313 w322]
                tunnel: [w312 w322] -> w292
                frame False {
                  n102 = call "MotionControl.vi"("Frequency (Hz) 3"=u32 650, "Motion Type"=enum16{"Linear", "Rotational"}."Linear", "Error In"=w320, "Distance"=w317, "Direction"=TRUE, "AirSAS Controls"=w313) -> ("Error Out"=w316:errorcluster, "output cluster"=w312:T1)  [unwired: 4 in]
                  n103 = property on="Slide" class="Slide (strict)"(error in=w316, "Value"=w315) -> (error out=w314:errorcluster)  [unwired: 1 in, 1 out]
                }
                frame True {
                }
              }
              n104 = Bundle By Name(cluster=w292, "Hardware.Height"=w291) -> (w299:T1)
            }
            n105 = call "Re-Init.vi"("Motion Control"=w261, "Enum"=enum16{"Circular", "Cylindrical", "Spiral"}."Cylindrical", "error in (no error)"=w260, "# lin. steps"=w257, "# rot. steps"=w258, "AirSAS Controls"=w263) -> ("error out"=w259:errorcluster, "output cluster"=w262:T1)  [unwired: 4 in]
          }
          frame "Spiral" {
            n106 = Unbundle By Name(w508) -> ("Vertical Min"=w496:dbl, "Vertical Max"=w495:dbl, "Vertical Step"=w494:dbl)
            n107 = call "InitTrack.vi"("AirSAS Controls in"=w506, "Vertical Min"=w496, "error in (no error)"=w505) -> ("AirSAS Controls out"=w504:T1, "output cluster"=w493:cluster{dbl, dbl, dbl}, "error out"=w502:errorcluster)  [unwired: 4 in]
            n108 = call "NumSteps.vi"("Step"=w494, "Stop"=w495, "Start"=w496) -> ("Numeric"=w497:dbl)  [unwired: 8 in]
            n109 = property on="Slide" class="Slide (strict)"(error in=w502, "Value"=w493) -> (error out=w501:errorcluster)  [unwired: 1 in, 1 out]
            n110 = for {
              N: w497 -> [w536]
              tunnel: w500 -> [w509]
              tunnel: w507 -> [w538]
              shift-right: [w510] -> w492
              shift-left: w504 -> [w542]
              tunnel: w503 -> [w537]
              shift-right: [w524] -> w499
              shift-left: w501 -> [w534]
              tunnel: w493 -> [w517]
              i -> [w513]
              n111 = Unbundle By Name(w509) -> ("Vertical Step"=w523:dbl, "Angular Stop"=w529:dbl, "Angular Start"=w526:dbl, "Angular Step"=w528:dbl)
              n112 = Decrement(x=w536) -> (x-1=w535:i32)
              n113 = Multiply(x=w528, y=w513) -> (x*y=w541:dbl)
              n114 = Add(x=w526, y=w541) -> (x+y=w527:dbl)
              n115 = Bundle By Name(cluster=w542, "Hardware.Angle"=w527) -> (w514:T1)
              n116 = Bundle(cluster=cluster{dbl, dbl, dbl} {-172.55422153679154, 17.21837893351085, -51.118830131082746} ("Gauge 2"), w526, w527, w529) -> (w540:cluster{dbl, dbl, dbl})
              n117 = property on="Gauge" class="Knob (strict)"(error in=w534, "Value"=w540) -> (error out=w533:errorcluster)  [unwired: 1 in, 1 out]
              n118 = for {
                N: w537 -> [w582]
                tunnel: w513 -> [w581]
                tunnel: w538 -> [w567]
                shift-right: [w566] -> w532
                shift-left: w514 -> [w568]
                shift-right: [w563] -> w531
                shift-left: w533 -> [w579]
                i -> [w580]
                # "air temp"
                # "file id"
                n119 = Multiply(x=w582, y=w581) -> (x*y=w584:i32)
                n120 = Increment(x=w580) -> (x+1=w583:i32)
                n121 = Unbundle By Name(w568) -> ("Port"=w574:dbl)
                n122 = Add(x=w584, y=w583) -> (x+y=w565:i32)
                n123 = To Long Integer(number=w574) -> (32bit integer=w575:i32)
                n124 = call "newTemp.vi"("port"=w575) -> ("Response String"=w573:string)  [unwired: 10 in]
                n125 = call "AcquireData.vi"("error in"=w579, "AirSAS Controls In"=w568) -> ("error out"=w578:errorcluster, "data"=w576:waveform(dbl), "AirSAS Controls Out"=w566:T1)  [unwired: 7 in]
                n126 = xnode "Match Regular Expression"("input string"=w573, "regular expression"="tmpr,....,") -> ("after match"=w571:string)  [unwired: 4 in, 4 out]
                n127 = property on="Acquired Data" class="WFGraph (strict)"(error in=w578, "Value"=w576) -> (error out=w577:errorcluster)  [unwired: 1 in, 1 out]
                n128 = call "Acoustic Save H5.vi"("Captured Data"=w576, "base path"=w567, "error in (no error)"=w577, "ID"=w565) -> ("error out"=w563:errorcluster)  [unwired: 7 in]
                n129 = Search/Split String(string=w571, search string/char (-)=",") -> (substring before match=w572:string)  [unwired: 1 in, 2 out]
                n130 = Fract/Exp String To Number(string=w572) -> (number=w564:dbl)  [unwired: 3 in, 1 out]
                n131 = call "CoordinateSave.vi"("Path"=w567, "Air Temperature"=w564, "Flight"=w565, "AirSAS Controls"=w566) -> ()  [unwired: 8 in]
              }
              n132 = Increment(x=w513) -> (x+1=w512:i32)
              n133 = Not Equal?(x=w535, y=w513) -> (x != y?=w515:bool)
              n134 = Add(x=w527, y=w528) -> (x+y=w530:dbl)
              n135 = Bundle("Angular Start"=w526, w530, "Angular Stop"=w529) -> (w525:T11)  [unwired: 1 in]
              n136 = Unbundle By Name(w509) -> ("Vertical Min"=w520:dbl, "Vertical Max"=w521:dbl, "Vertical Step"=w518:dbl)
              n137 = Multiply(x=w512, y=w518) -> (x*y=w519:dbl)
              n138 = Add(x=w520, y=w519) -> (x+y=w522:dbl)
              n139 = Bundle(cluster=w517, w520, w522, w521) -> (w516:cluster{dbl, dbl, dbl})
              n140 = case shown="True" w515 {
                tunnel: w532 -> [w544 w559]
                tunnel: w531 -> [w543 w558]
                tunnel: w528 -> [_ w556]
                tunnel: w525 -> [_ w555]
                tunnel: [w543 w553] -> w524
                tunnel: w523 -> [_ w551]
                tunnel: w516 -> [_ w550]
                tunnel: [w544 w545] -> w511
                frame False {
                }
                frame True {
                  # "clockwise"
                  n141 = call "MotionControl.vi"("Frequency (Hz) 3"=u32 1000, "Motion Type"=enum16{"Linear", "Rotational"}."Rotational", "Error In"=w558, "Distance"=w556, "Direction"=FALSE, "AirSAS Controls"=w559) -> ("Error Out"=w557:errorcluster, "output cluster"=w552:T1)  [unwired: 4 in]
                  n142 = property on="Gauge" class="Knob (strict)"(error in=w557, "Value"=w555) -> (error out=w554:errorcluster)  [unwired: 1 in, 1 out]
                  n143 = call "MotionControl.vi"("Frequency (Hz) 3"=u32 650, "Motion Type"=enum16{"Linear", "Rotational"}."Linear", "Error In"=w554, "Distance"=w551, "Direction"=TRUE, "AirSAS Controls"=w552) -> ("Error Out"=w547:errorcluster, "output cluster"=w545:T1)  [unwired: 4 in]
                  n144 = property on="Slide" class="Slide (strict)"(error in=w547, "Value"=w550) -> (error out=w553:errorcluster)  [unwired: 1 in, 1 out]
                }
              }
              n145 = Bundle By Name(cluster=w511, "Hardware.Height"=w522) -> (w510:T1)
            }
            n146 = call "Re-Init.vi"("Motion Control"=w500, "Enum"=enum16{"Circular", "Cylindrical", "Spiral"}."Spiral", "error in (no error)"=w499, "# rot. steps"=w497, "AirSAS Controls"=w492) -> ("error out"=w498:errorcluster, "output cluster"=w491:T1)  [unwired: 5 in]
          }
        }
      }
      event "stop": Value Change {
        n147 = event-data() -> ()  [unwired: 1 in, 6 out]
      }
    }
  }
  "error out" <- w15
  "AirSAS Controls 2" <- w7
